vi "Formater tab historique.vi"() -> (0 "tab histo reformaté":string[](array[string]))   [LabVIEW 2020]
doc: "Met en forme le n° de valve déjà emballée :\n- si pas un retour (col 5 =0), n° inchangé (ex: 112105740008090001)\n- si pas un retour (col 5 >0), n° concaté avec n° retour (ex: 112105740008090001R2)"
uses:
  Modules/FS/60_FS_Controles/60_FS_SetGet.ctl
panel:
  out "tab pcs emballées historique":string[][](array[string])=[["112101230108120020"], ["112101230108120021"], ["112101230108120022"], ["112101230108120023"]]
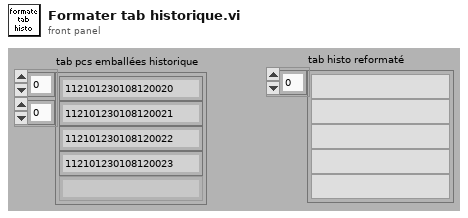
[diagram p1: front panel]
types:
  T1 = typedef "60_FS_SetGet.ctl" = enum16{"set", "get"}
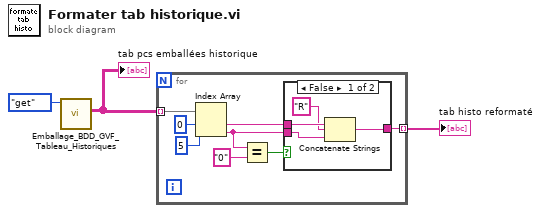
[diagram p0: block diagram]
diagram:
  n1 = call "Emballage_BDD_GVF_Tableau_Historiques.vi"("SetGet"=60_FS_SetGet."get") -> ("Tableau historique OUT"=w2:string[][])  [unwired: 9 in, 1 out]
  "tab pcs emballées historique" <- w2
  n2 = for {
    tunnel: w2 -> [w11] mode=indexing
    tunnel: [w5] -> w3 mode=indexing
    n3 = Index Array(array=w11, index #1=0 ("indice"), index #2=5 ("indice")) -> (element #1=w6:string, element #2=w4:string)
    n4 = Equal?(x=w4, y="0") -> (x = y?=w7:bool)
    n5 = case shown="False" w7 {
      tunnel: w6 -> [w14 w16]
      tunnel: [w15 w16] -> w5
      tunnel: w4 -> [w12 _]
      frame False {
        n6 = Concatenate Strings(w14, "R" ("y"), w12) -> (w15:string)
      }
      frame True {
      }
    }
  }
  "tab histo reformaté" <- w3
